vi "CTRE_Phoenix_CANdle_LarsonAnimation.vi"(0 "CTRE_CANdle_DeviceRef":T3, 1 "Size":i32=2, 2 "Bounce Mode":T1 items=["Front", "Center", "Back"], 5 "Speed":dbl=1.0 min=0.0 max=1.0 step=0.0001, 7 "Num LEDs":i32=-1, 9 "LED Color":T2, 11 "error in":errorcluster) -> (4 "CTRE_CANdle_DeviceRef":T3, 15 "error out":errorcluster)   [LabVIEW 2020]
doc: "Animation that sends a pocket of light across the LED strip.\n\n<b>Speed</b> adjust the speed at which the animation runs. Valid values range from 0 to 1 where 1 is the fastest animation speed.\n\n<b>Num LEDs</b> defines the total number of LEDs to use for the animation.\n\n<b>LED Color</b> is the RGB(W) value of the color to illuminate.\n\n<b>Size</b> is the number of LEDs in the pocket of light that travels along the LED strip.\n\n<b>Bounce Mode</b> defines which LED in the pocket of light is the poing that bounces at the end of the LED strip."
uses:
  <vilib>/Rock Robotics/WPI/ThirdParty/Phoenix-LabVIEW/CANdle/Controls/CTRE_Phoenix_CANdle_DeviceRef.ctl
  <vilib>/Rock Robotics/WPI/ThirdParty/Phoenix-LabVIEW/CANdle/Controls/CTRE_Phoenix_CANdle_LEDColor.ctl
  <vilib>/Rock Robotics/WPI/ThirdParty/Phoenix-LabVIEW/CANdle/Controls/CTRE_Phoenix_CANdle_AnimationLarsonBounce.ctl
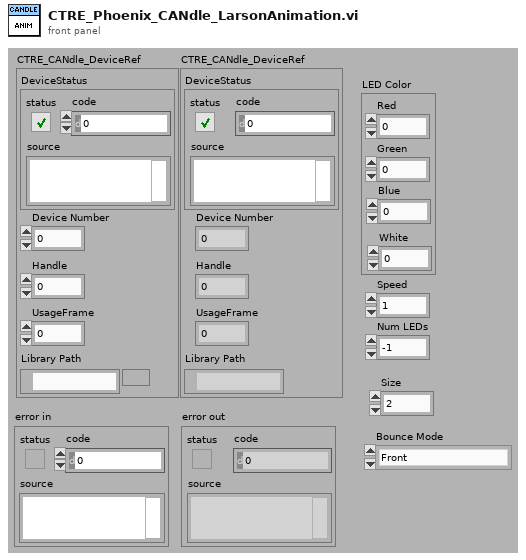
[diagram p1: front panel]
types:
  T1 = typedef "CTRE_Phoenix_CANdle_AnimationLarsonBounce.ctl" = u16
  T2 = typedef "CTRE_Phoenix_CANdle_LEDColor.ctl" = cluster{"Red":u8, "Green":u8, "Blue":u8, "White":u8}
  T3 = typedef "CTRE_Phoenix_CANdle_DeviceRef.ctl" = cluster{"DeviceStatus":errorcluster, "Device Number":u8, "Handle":u64, "UsageFrame":u32, "Library Path":path}
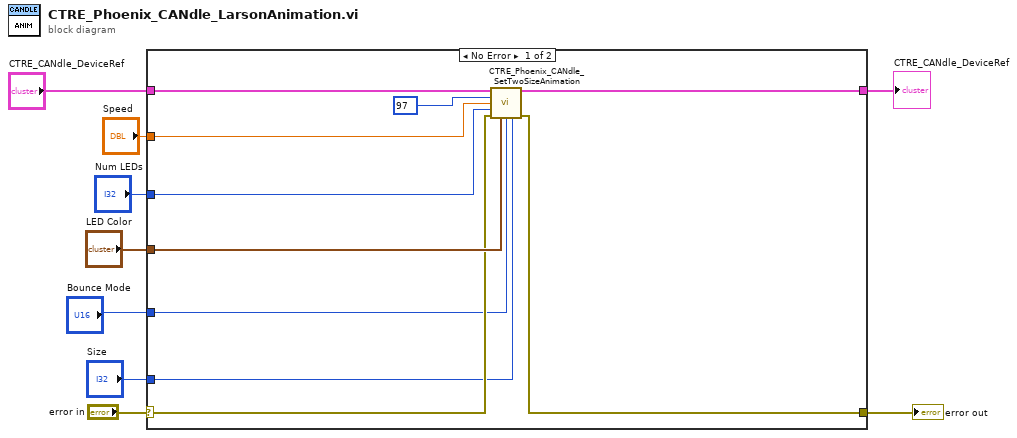
[diagram p0: block diagram]
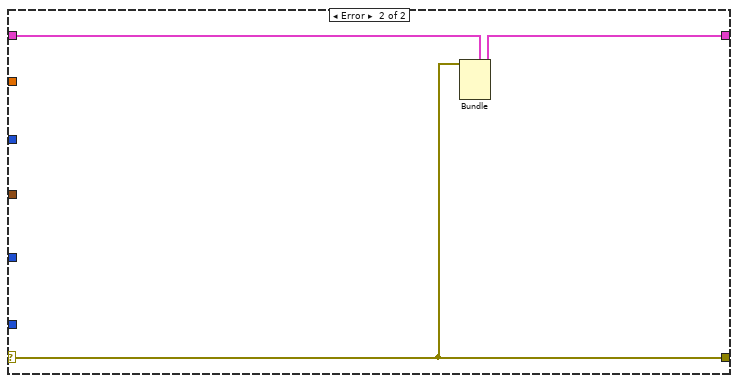
[diagram p2: hidden frame]
diagram:
  n1 = case shown="No Error" "error in" {
    selector: "error in" -> [w13 w21]
    tunnel: "CTRE_CANdle_DeviceRef" -> [w19 w22]
    tunnel: [w12 w21] -> w9
    tunnel: [w18 w20] -> w6
    tunnel: "LED Color" -> [w17 _]
    tunnel: "Speed" -> [w15 _]
    tunnel: "Num LEDs" -> [w14 _]
    tunnel: "Size" -> [w11 _]
    tunnel: "Bounce Mode" -> [w10 _]
    frame No Error {
      n2 = call <vilib>:"CTRE_Phoenix_CANdle_SetTwoSizeAnimation.vi"("CTRE_CANdle_DeviceRef"=w19, "idx"=97, "speed"=w15, "numLED"=w14, "error in"=w13, "LED Color"=w17, "direction"=w10, "size"=w11) -> ("CTRE_CANdle_DeviceRef"=w18:T3, "error out"=w12:errorcluster)  [unwired: 6 in]
    }
    frame Error {
      n3 = Bundle(cluster=w22, "DeviceStatus"=w21) -> (w20:T3)  [unwired: 4 in]
    }
  }
  "error out" <- w9
  "CTRE_CANdle_DeviceRef" <- w6
